vi "Coordinate2Address.vi"(1 "Column":i32, 2 "Row":i32) -> (0 "Address":string)   [LabVIEW 2026, in "XCel Report Engine.lvlib"]
uses:
  XCel Report Engine.lvlib
  C:/Users/m.santucci/Documents/ChatGPT/LV_REPORT_ENGINE/.net/src/XCelReportEngine/bin/Release/net48/XCelReportEngine.dll
  .net/src/XCelReportEngine/bin/Release/net48/XCelReportEngine.dll
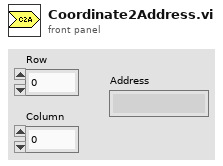
[diagram p1: front panel]
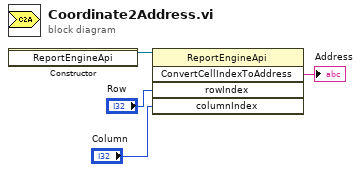
[diagram p0: block diagram]
diagram:
  n1 = constructor class="ReportEngineApi"() -> (reference out=w4:refnum<k24>)  [unwired: 3 in, 2 out]
  n2 = invoke class="ReportEngineApi" method="ConvertCellIndexToAddress"(reference=w4, "rowIndex"="Row", "columnIndex"="Column") -> ("ConvertCellIndexToAddress"=→"Address":string)  [unwired: 2 in, 4 out]
